vi "Dummy VI.vi"() -> ()   [LabVIEW 2015]
panel:
  in  "Reference":void[](array[numeric])
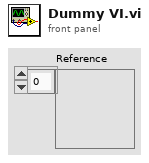
[diagram p1: front panel]
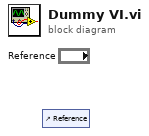
[diagram p0: block diagram]
diagram:
  n1 = control-ref of="Reference"() -> ()  [unwired: 1 out]
